vi "ManagerClose.vi"(8 "error in":errorcluster, 11 "Manager In":u64 caption="Device In") -> (0 "error out":errorcluster)   [LabVIEW 2012, in "Phidget Manager.lvlib"]
doc: "${Accelerometer:CloseHeader}"
uses:
  <instrlib>/Phidgets/Phidget Manager/Phidget Manager.lvlib
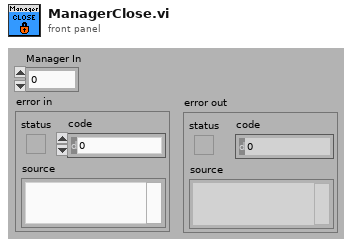
[diagram p1: front panel]
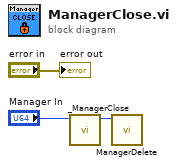
[diagram p0: block diagram]
diagram:
  n1 = call <instrlib>:"_ManagerClose.vi"("Device In"="Manager In") -> ("Device Out"=w1:u64)  [unwired: 9 in, 1 out]
  n2 = call <instrlib>:"ManagerDelete.vi"("Device In"=w1) -> ()  [unwired: 10 in, 1 out]
  "error out" <- "error in"
